vi "DSF.Engine.Plugin.Set Transceiver Threads.vi"(10 "Transceivers":refnum<class "DSF.Engine.Transceiver Thread.lvclass">[](array[class]), 11 "Plugin in":refnum<class "DSF.Engine.Plugin.lvclass">) -> (3 "Plugin out":refnum<class "DSF.Engine.Plugin.lvclass">)   [LabVIEW 2017, in "DSF.Engine.lvlib" / "DSF.Engine.Plugin.lvclass"]
uses:
  DSF.Engine.Plugin.lvclass
  Transceiver/DSF.Engine.Transceiver Thread.lvclass
  DSF.Engine.Plugin.lvclass/DSF.Engine.Plugin.ctl
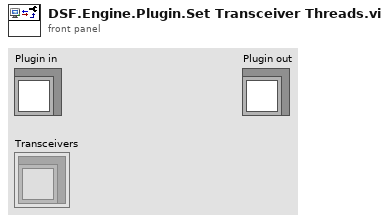
[diagram p1: front panel]
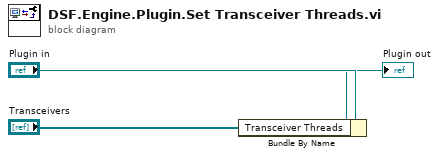
[diagram p0: block diagram]
diagram:
  n1 = Bundle By Name(cluster="Plugin in", "Transceiver Threads"="Transceivers") -> (→"Plugin out":refnum<class "DSF.Engine.Plugin.lvclass">)
